vi "ADI_IMU_ADIS16470_FGV.vi"(0 "ADI IMU DevRef":T2, 1 "Operation":enum16{"set", "get", "set reset"}(ring), 2 "Sensor Ready?":bool, 5 "Reset":bool, 7 "IMU Data":T1, 9 "IMU Angles":T4, 11 "error in":errorcluster) -> (4 "ADI IMU DevRef Out":T2, 6 "Reset Out":bool, 8 "IMU Data":T1, 10 "IMU Angles Out":T4, 13 "Sensor Ready Out":bool, 15 "error out":errorcluster)   [LabVIEW 2018, in "ADIS16470_IMU.lvlib"]
uses:
  ADIS16470_IMU.lvlib
  ADI_IMU_ADIS16470_IMUDevRef.ctl
  <vilib>/Rock Robotics/SystemInterfaces/spilib/spi_bus.ctl
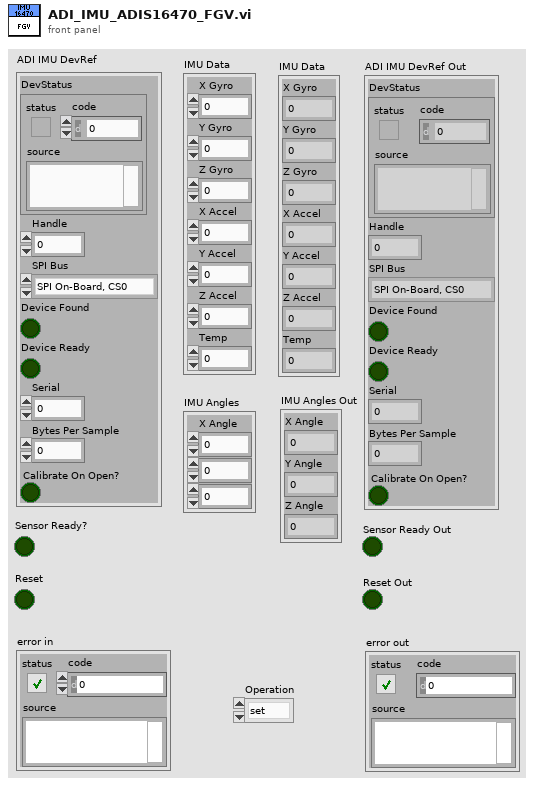
[diagram p1: front panel]
types:
  T1 = cluster{"X Gyro":dbl, "Y Gyro":dbl, "Z Gyro":dbl, "X Accel":dbl, "Y Accel":dbl, "Z Accel":dbl, "Temp":dbl}
  T2 = typedef "ADIS16470_IMU.lvlib/ADI_IMU_ADIS16470_IMUDevRef.ctl" = cluster{"DevStatus":errorcluster, "Handle":i32, "SPI Bus":T3, "Device Found":bool, "Device Ready":bool, "Serial":u16, "Bytes Per Sample":u16, "Calibrate On Open?":bool}
  T3 = typedef "spi_bus.ctl" = enum16{"SPI On-Board, CS0", "SPI On-Board, CS1", "SPI On-Board, CS2", "SPI On-Board, CS3", "SPI MXP", "Invalid"}
  T4 = cluster{"X Angle":dbl, "Y Angle":dbl, "Z Angle":dbl}
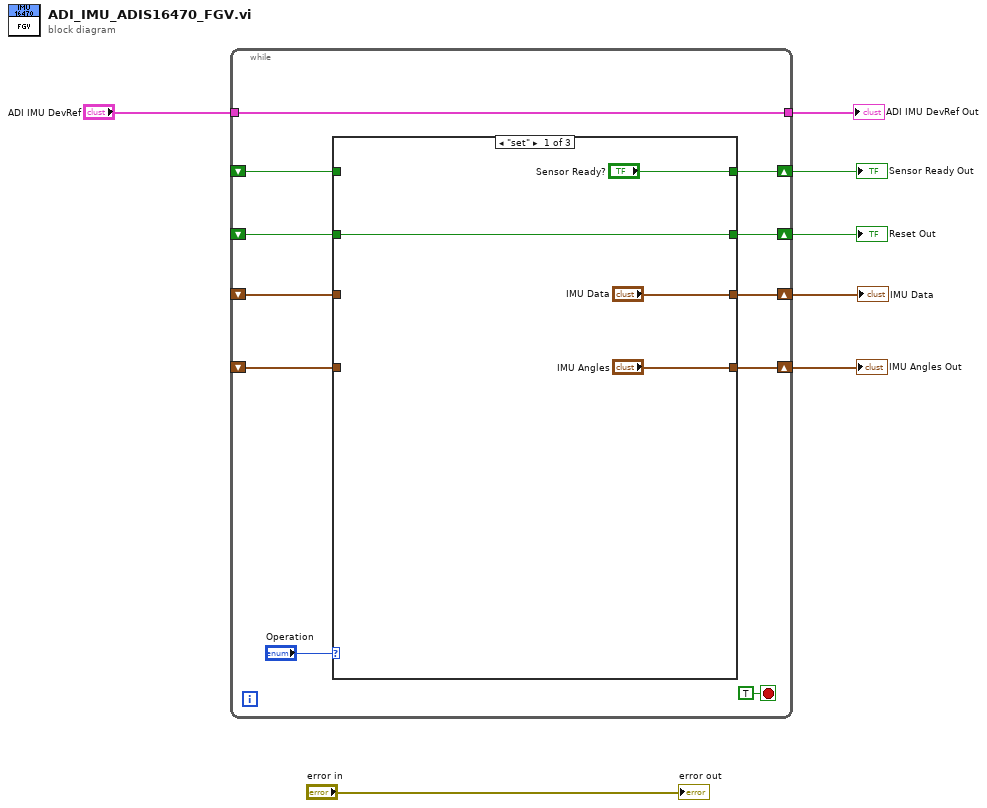
[diagram p0: block diagram]
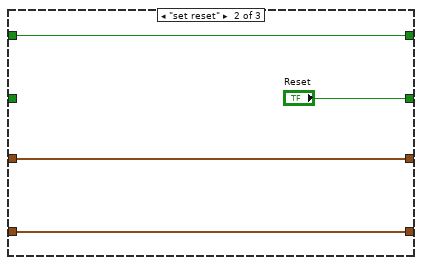
[diagram p2: hidden frame]
diagram:
  n1 = while {
    shift-right: [w16] -> w7
    shift-left: _ -> [w10]
    shift-right: [w15] -> w4
    shift-left: _ -> [w11]
    tunnel: "ADI IMU DevRef" -> [w14]
    tunnel: [w14] -> w5
    shift-right: [w13] -> w3
    shift-left: _ -> [w12]
    shift-right: [w8] -> w6
    shift-left: _ -> [w9]
    stop <- TRUE stop-if-true
    n2 = case shown="\"set\"" "Operation" {
      tunnel: [w20 "Reset" w28] -> w16
      tunnel: ["IMU Data" w24 w29] -> w15
      tunnel: ["IMU Angles" w25 w30] -> w13
      tunnel: w12 -> [_ w25 w30]
      tunnel: w11 -> [_ w24 w29]
      tunnel: w10 -> [w20 _ w28]
      tunnel: ["Sensor Ready?" w23 w27] -> w8
      tunnel: w9 -> [_ w23 w27]
      frame "set" {
      }
      frame "set reset" {
      }
      frame "get", Default {
      }
    }
  }
  "Reset Out" <- w7
  "Sensor Ready Out" <- w6
  "IMU Angles Out" <- w3
  "ADI IMU DevRef Out" <- w5
  "IMU Data" <- w4
  "error out" <- "error in"
